vi "LuaVIEW Register Private Function Directory.vi"(5 "LuaVIEW reference in":T1, 7 "base path":path, 11 "error in (no error)":errorcluster) -> (6 "LuaVIEW reference out":T1, 15 "error out":errorcluster)   [LabVIEW 2012]
doc: "Tries to register all VIs ending in \"_lua.vi\" in a directory or llb and, recursively, in any subdirectories or llbs, or, alternatively, inside a built executable as private LuaVIEW functions with the provided LuaVIEW state."
uses:
  typedefs/t_LuaVIEW Reference.ctl
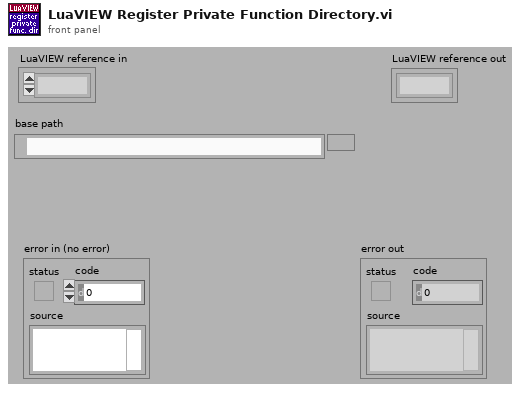
[diagram p1: front panel]
types:
  T1 = typedef "t_LuaVIEW Reference.ctl" = refnum<k1>
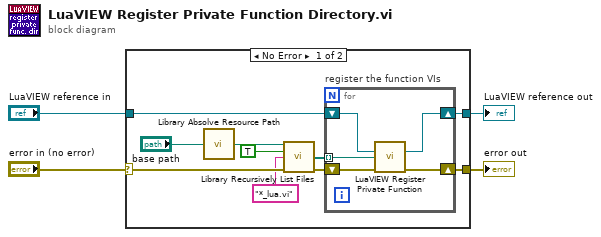
[diagram p0: block diagram]
diagram:
  n1 = case shown="No Error" "error in (no error)" {
    selector: "error in (no error)" -> [w12 w21]
    tunnel: [w11 w21] -> w4
    tunnel: "LuaVIEW reference in" -> [w6 w20]
    tunnel: [w5 w20] -> w1
    frame No Error {
      n2 = call "Library Absolve Resource Path.vi"("path in"="base path") -> ("absolved path"=w9:path)  [unwired: 14 in]
      n3 = call "Library Recursively List Files.vi"("root directory"=w9, "enter llbs? (no)"=TRUE, "pattern (none)"="*_lua.vi" ("pattern"), "error in (no error)"=w12) -> ("file list"=w14:path[], "error out"=w13:errorcluster)  [unwired: 9 in, 1 out]
      n4 = for "register the function VIs" {
        shift-right: [w18] -> w11
        shift-left: w13 -> [w19]
        tunnel: w14 -> [w17] mode=indexing
        shift-right: [w15] -> w5
        shift-left: w6 -> [w16]
        n5 = call "LuaVIEW Register Private Function.vi"("LuaVIEW reference in"=w16, "function VI path"=w17, "error in (no error)"=w19) -> ("LuaVIEW reference out"=w15:T1, "error out"=w18:errorcluster)  [unwired: 11 in]
      }
    }
    frame Error {
    }
  }
  "error out" <- w4
  "LuaVIEW reference out" <- w1
